vi "NI GetWaveform.vi"(0 "Acq ID In":refnum<k15>, 1 "Num Samps":i32=1000, 2 "Rcv Ring":i32, 3 "Reverse?":bool, 4 "Num Segs":i32=1, 5 "Motion Settings":T1={"No Motion?"=FALSE, "Motion System"=enum."NI 735x", "Motion Bd ID"=1, "Motion Profile"="SMAC1", "# Axis"=1, "Reverse Z axis?"=TRUE, "SMAC Axis"=0, "scan pair"=enum."y-(x) scan", "RT fps"=6.0, "Steps per mm"=[1000, 1000, 1000, 1000], "Motor Parameters"={"velocity ct/s"=[10000.0, 10000.0, 10000.0, 50000.0], "accel ct/s^2"=[50000.0, 50000.0, 50000.0, 200000.0]}, "One Way Scan"=FALSE, "Reverse One Way Scan"=FALSE, "Global Position (mm)"=[], "Plane"=0, "Distance between\nscan lines (um)"=0.0, "Distance between\nscan planes (um)"=0.0, "number of scan planes"=1, "Total steps in line"=0, "Xtra plane\ndistance  (um)"=100, "Xtra planes "=1, "Add Axis"=FALSE, "overshoot cts"=200, "BKPT Shift"=0, "Scan Start Time (ms)"=0, "ESP VISA"="GPIB::1::INSTR", "3rd Axis"=1, "GL Ref Out"=refnum, "Galil Address"=""} {"3rd Axis" items=["x", "y", "z", "w"]; "Xtra planes" min=1; "Xtra plane\ndistance  (um)" min=0; "Distance between\nscan planes (um)" format="%.2f"; "Distance between\nscan lines (um)" format="%.2f"; "SMAC Axis" items=["None"=0, "Axis 1"=1, "Axis 2"=2, "Axis 3"=3, "Axis 4"=4, "Axis 5"=5, "Axis 6"=6, "Axis 7"=7, "Axis 8"=8, "Vector Space 1"=17, "Vector Space 2"=18, "Vector Space 3"=19, "Vector Space 4"=20]; "Motion Bd ID" min=1 max=32 step=1}, 6 "Read Method":u16(ring) items=["Not used", "RT Read", "RT Save", "Scaled Voltage"], 7 "Channel":i32, 9 "error in":errorcluster, 10 "timeout":dbl=1.0, 11 "File Array":string[](array[string])=["blank"], 12 "Digitizer Settings":T5={"Digitizer delay (us) "=0.0, "rf points per line"=2048, "lines per plane"=128, "Samp Rate (Hz)"=100000000.0, "Additional dig delay (us)"=0.0, "Voltage Scale"=0.4, "Pre-Looks"=0, "Offset delay (us)"=0.0, "bits A/D"=8, "Avg Num"=1, "DigTimeOut"=5.0, "Rel Dig Delay"=0.0, "Dig Ch"=0, "LeCroyCluster"={"LeCroy Channels"=[TRUE, FALSE, FALSE, FALSE], "LC read pt offset"=0.0, "Sweep Avg"=FALSE}, "Main Digitizer"=enum."NI Digitizer", "Dig Config"=enum."Single channel", "Digitizer ID Cluster"={"Acqiris/Alazar/SP ID"=[], "NI Instr Handles"=[], "LeCroy VISA"="", "GaGe Handle"={"Handle"=0, "Sample size"=0, "Resolution"=0, "Offset"=0, "Channels"=0, "Boards"=0}, "ATS Ref"="ATS9350", "Acqiris Address"=["PCI::INSTR0"], "ADQRef"=refnum, "adq_cu_ptr"=refnum}, "Trigger Settings"={"Trig Source"=1, "Trig Coupling"=0, "Trig Slope"=0, "Level (mV)"=1500.0}, "Bulk Acq"=FALSE, "Bulk Start Indexes"=[], "Data Ref RF"=refnum, "NI ID/Channel"=[], "Total Dig CH"=1, "Xtra Ann Trig delay (us)"=10.0, "Fix Z Delay?"=FALSE, "One Way Transmission?"=FALSE, "Data Ref Log"=refnum} {"Trigger Settings"."Trig Slope" items=["Positive", "Negative"]; "Trigger Settings"."Level (mV)" format="%.2f"; "Trigger Settings"."Trig Coupling" items=["DC 1 MOhm", "AC 1 MOhm", "DC 50 Ohm", "AC 50 Ohm"]; "Trigger Settings"."Trig Source" items=["Chan 1", "External"]; "Rel Dig Delay" format="%.2f"; "DigTimeOut" format="%.2f"; "Avg Num" min=1; "Offset delay (us)" format="%.2f"; "Additional dig delay (us)" format="%.2f"; "Digitizer delay (us)" format="%.2f"}, 13 "Start Record":i32) -> (14 "Acq ID Out":refnum<k15>, 15 "Gain Array":T9(array[cluster]), 17 "Acquired Waveform16 bit":i8[][](array[numeric]), 18 "Acquired Waveform16 bit 2":i8[][](array[numeric]), 19 "error out":errorcluster)   [LabVIEW 2022 SP3]
uses:
  -DigitizerRoutines/DigitizerSettings.ctl
  -DigitizerRoutines/Digitizer.ctl
  -DigitizerRoutines/DigConfig.ctl
  -DigitizerRoutines/DigitizerID.ctl
  C:/Windows/System32/ADQAPI_dotNet_helper.dll
  Motion Controllers/NI_controller/-NI_MotionRoutines/MotionParameters.ctl
  Motion Controllers/NI_controller/-NI_MotionRoutines/MotionSys.ctl
  Motion Controllers/-MotionRoutines/ScanAxis.ctl
  Motion Controllers/-MotionRoutines/3rdAxis.ctl
  <instrlib>/niScope/Acquire/Fetch/niScope Multi Fetch Binary 8.vi
  -ScanSystem/DataHandling/ReverseDataI8.vi
  Motion Controllers/-MotionRoutines/MotionGlobals.vi
panel:
  # "Mujst convert data at output for Integers"
  # "1-D and 2-D B scan settings"
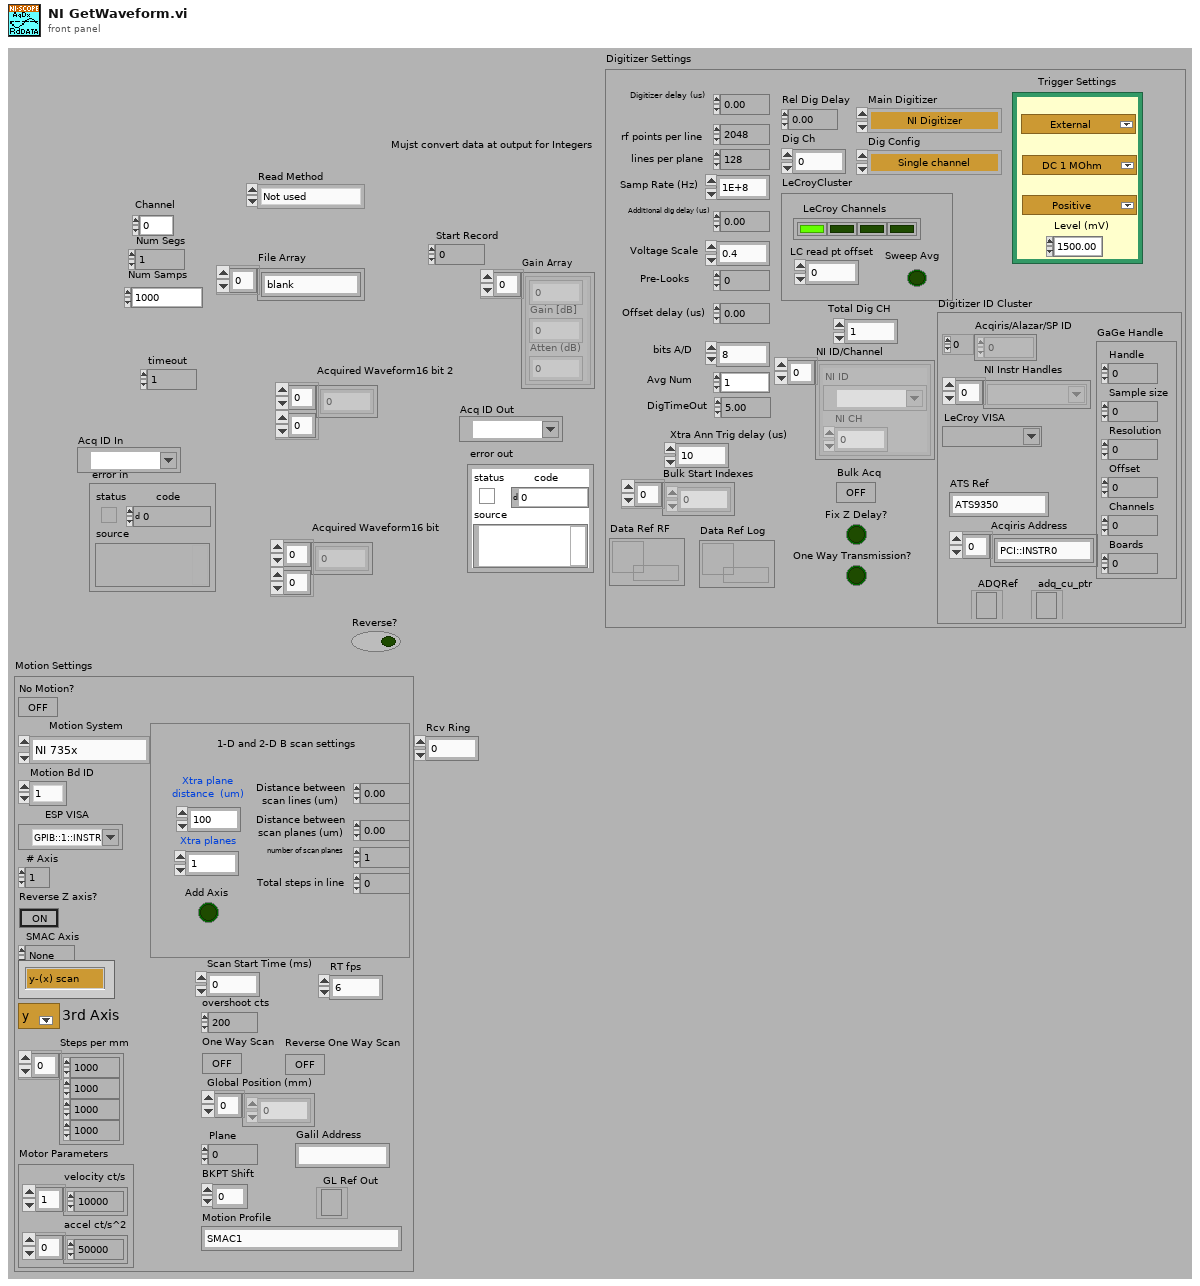
[diagram p1: front panel]
types:
  T1 = typedef "MotionParameters.ctl" = cluster{"No Motion?":bool, "Motion System":T2, "Motion Bd ID":u8, "Motion Profile":string, "# Axis":i8, "Reverse Z axis?":bool, "SMAC Axis":u16, "scan pair":T3, "RT fps":sgl, "Steps per mm":i32[], "Motor Parameters":cluster{"velocity ct/s":dbl[], "accel ct/s^2":dbl[]}, "One Way Scan":bool, "Reverse One Way Scan":bool, "Global Position (mm)":dbl[], "Plane":i32, "Distance between\nscan lines (um)":sgl, "Distance between\nscan planes (um)":sgl, "number of scan planes":i32, "Total steps in line":i32, "Xtra plane\ndistance  (um)":i32, "Xtra planes ":i32, "Add Axis":bool, "overshoot cts":i32, "BKPT Shift":i32, "Scan Start Time (ms)":u32, "ESP VISA":refnum<visa-resource-name>, "3rd Axis":T4, "GL Ref Out":refnum<k7>, "Galil Address":string}
  T2 = typedef "MotionSys.ctl" = enum16{"MM3000", "NI 735x", "Newport ESP", "No Motion Card", "Galil"}
  T3 = typedef "ScanAxis.ctl" = enum16{"y-(x) scan", "x-(y) scan", "z-(x) scan", "z-(y) scan", "y-(z) scan", "x-(z) scan", "w-(x) scan", "w-(y) scan", "w-(z) scan", "x-(w) scan", "y-(w) scan", "z-(w) scan"}
  T4 = typedef "3rdAxis.ctl" = u16
  T5 = typedef "DigitizerSettings.ctl" = cluster{"Digitizer delay (us) ":dbl, "rf points per line":i32, "lines per plane":i32, "Samp Rate (Hz)":dbl, "Additional dig delay (us)":dbl, "Voltage Scale":dbl, "Pre-Looks":i32, "Offset delay (us)":dbl, "bits A/D":i8, "Avg Num":i32, "DigTimeOut":sgl, "Rel Dig Delay":sgl, "Dig Ch":i32, "LeCroyCluster":cluster{"LeCroy Channels":bool[], "LC read pt offset":dbl, "Sweep Avg":bool}, "Main Digitizer":T6, "Dig Config":T7, "Digitizer ID Cluster":T8, "Trigger Settings":cluster{"Trig Source":u16, "Trig Coupling":u16, "Trig Slope":u16, "Level (mV)":dbl}, "Bulk Acq":bool, "Bulk Start Indexes":i32[], "Data Ref RF":refnum<data-value>, "NI ID/Channel":cluster{"NI ID":refnum<k15>, "NI CH":i32}[], "Total Dig CH":i32, "Xtra Ann Trig delay (us)":dbl, "Fix Z Delay?":bool, "One Way Transmission?":bool, "Data Ref Log":refnum<data-value>}
  T6 = typedef "Digitizer.ctl" = enum16{"Acqiris Digitizer", "NI Digitizer", "LeCroy", "GaGe", "AlazarTech", "No Digitizer", "Teledyne"}
  T7 = typedef "DigConfig.ctl" = enum16{"Single channel", "2 Chans w/ 2 Acqiris", "2 Chans w/ 1 Acqiris", "5-CH Pulser New", "5-CH pulser w/ ann array", "5-pass style ann array", "Empty"}
  T8 = typedef "DigitizerID.ctl" = cluster{"Acqiris/Alazar/SP ID":u32[], "NI Instr Handles":refnum<k15>[], "LeCroy VISA":refnum<visa-resource-name>, "GaGe Handle":cluster{"Handle":u32, "Sample size":u32, "Resolution":i32, "Offset":i32, "Channels":u32, "Boards":u32}, "ATS Ref":string, "Acqiris Address":string[], "ADQRef":refnum<k24>, "adq_cu_ptr":refnum<k24>}
  T9 = cluster{sgl, "Gain [dB]  ":sgl, "Atten (dB)":sgl}[]
  T10 = cluster{"actualSamples":i32, "absoluteInitialX":dbl, "relativeInitialX":dbl, "xIncrement":dbl, "offset":dbl, "gain":dbl, "reserved1":dbl, "reserved2":dbl}[]
  T11 = cluster{"actualSamples":i32, "absoluteInitialX":dbl, "relativeInitialX":dbl, "xIncrement":dbl, "offset":dbl, "gain":dbl, "reserved1":dbl, "reserved2":dbl}
  T12 = cluster{sgl, "Gain [dB]  ":sgl, "Atten (dB)":sgl}
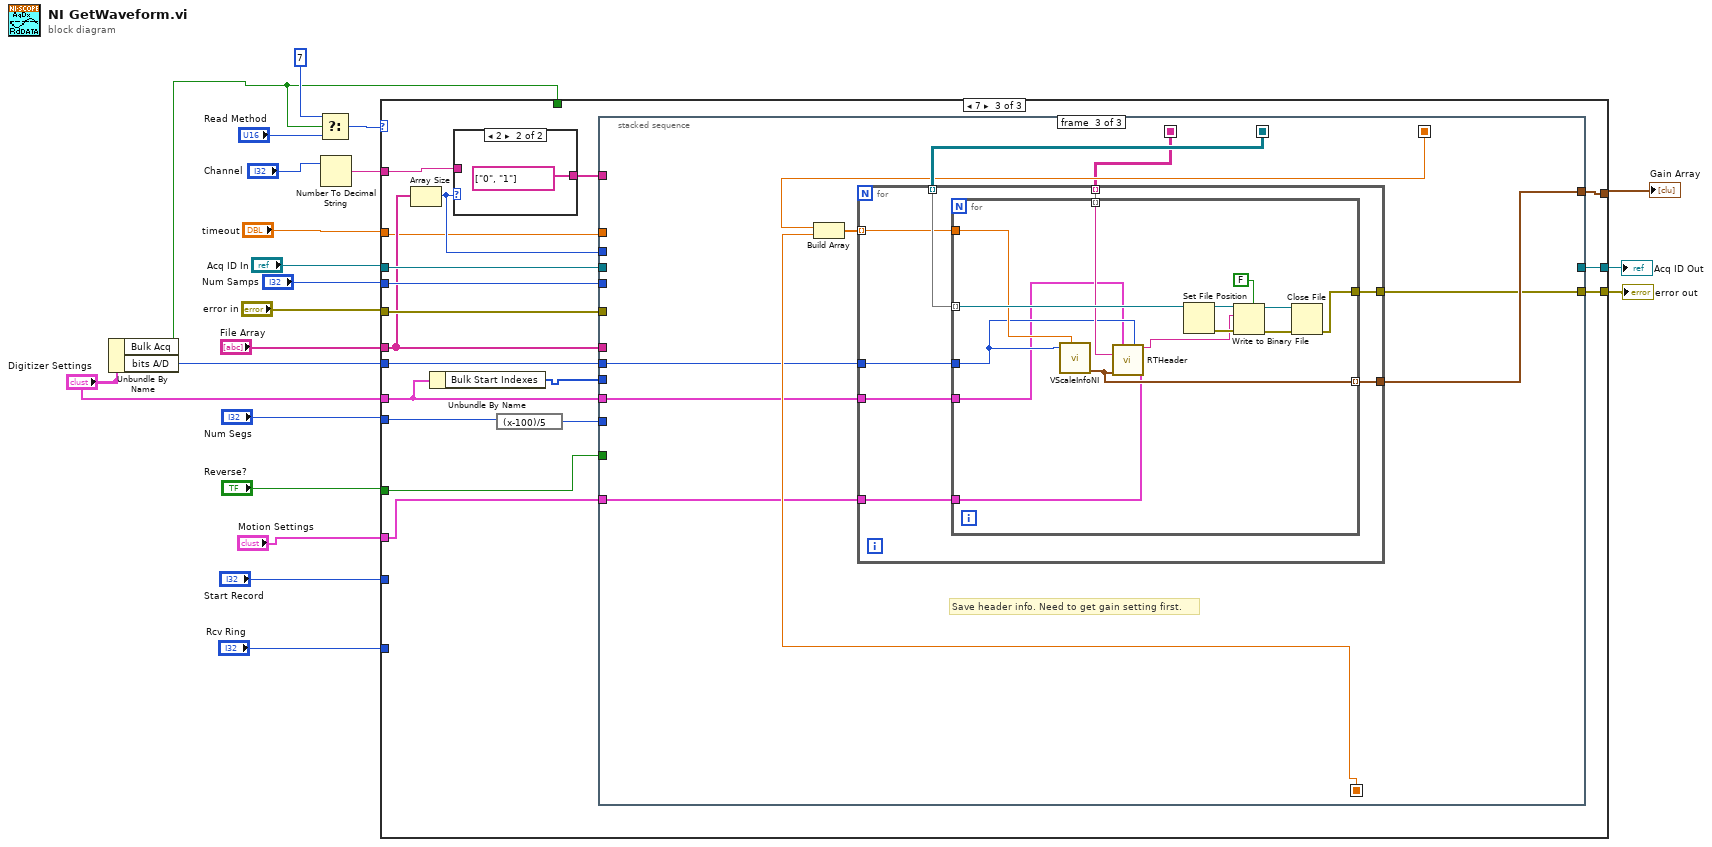
[diagram p0: block diagram]
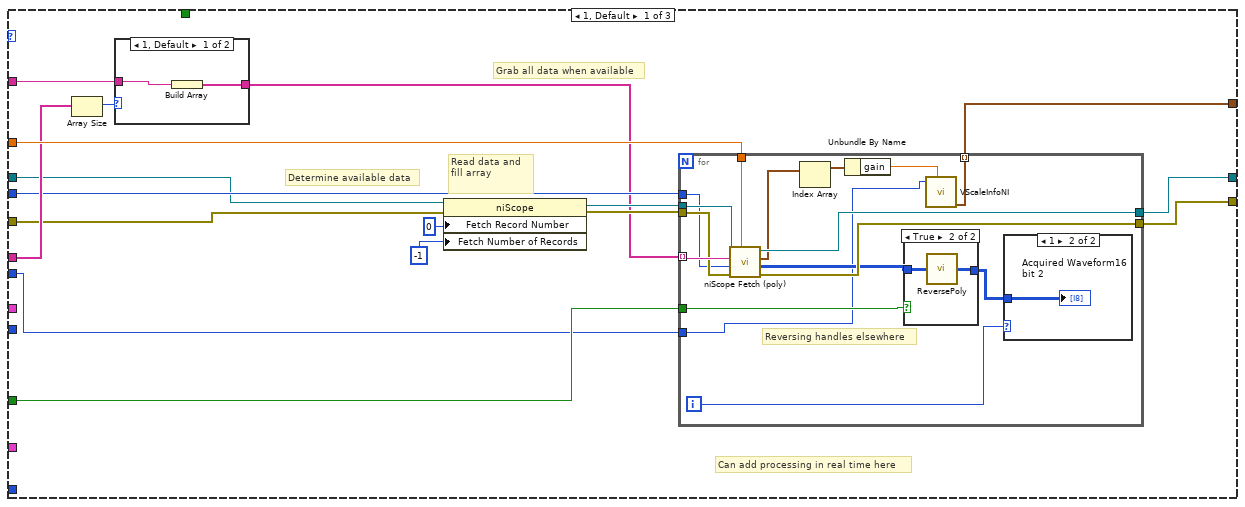
[diagram p2: hidden frame]
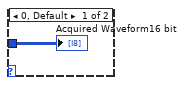
[diagram p3: hidden frame]
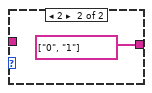
[diagram p5: hidden frame]
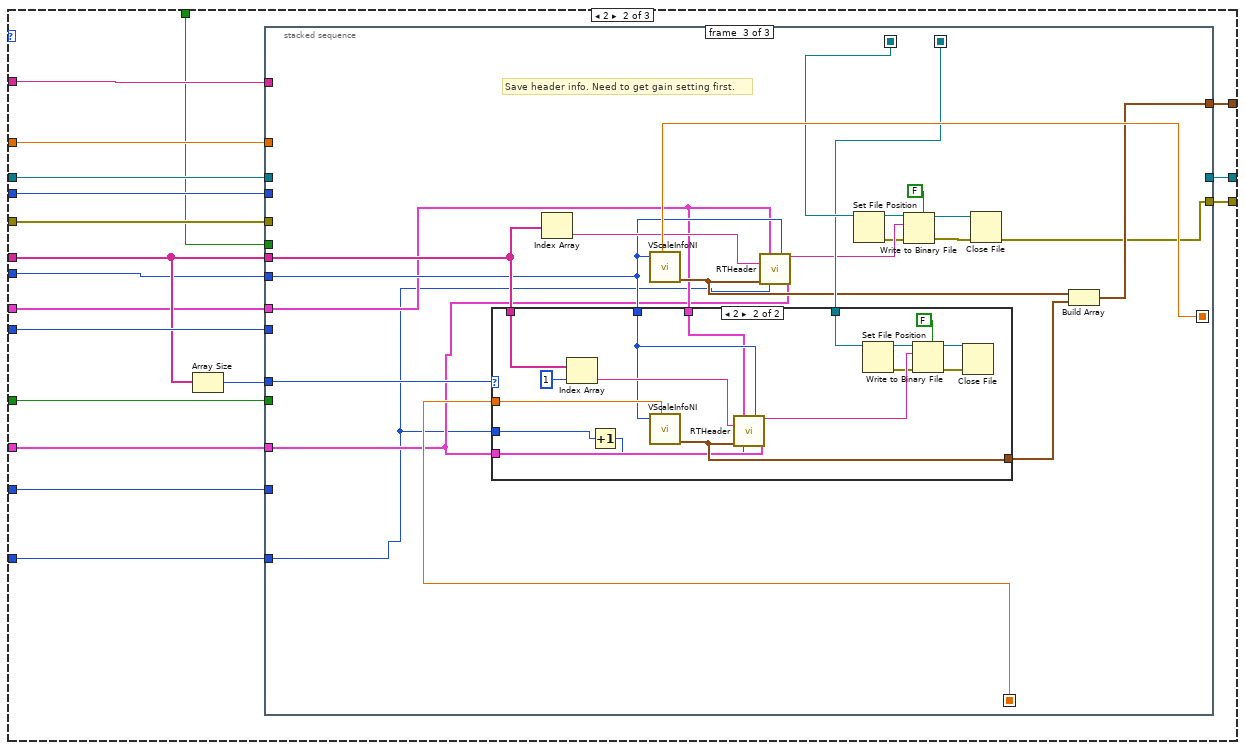
[diagram p6: hidden frame]
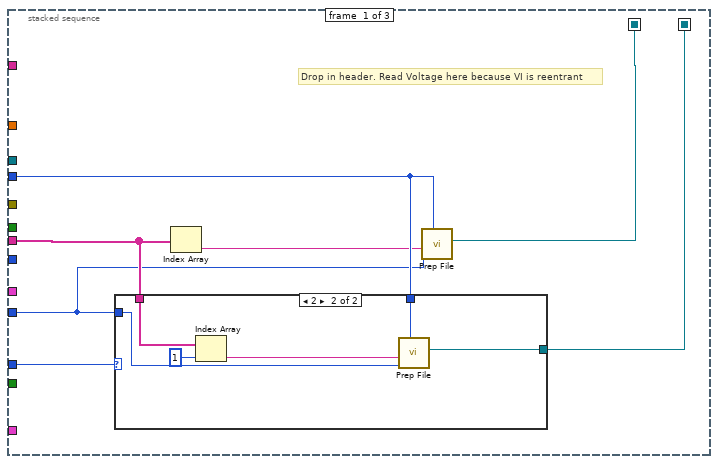
[diagram p7: hidden frame]
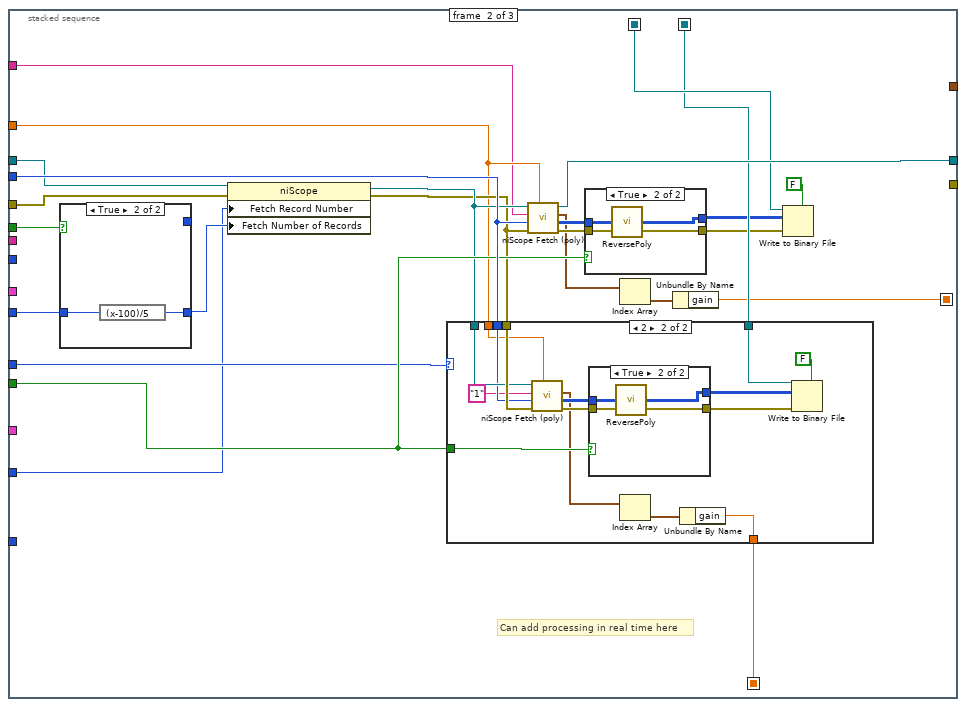
[diagram p9: hidden frame]
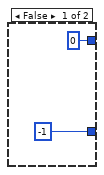
[diagram p13: hidden frame]
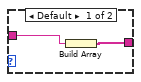
[diagram p15: hidden frame]
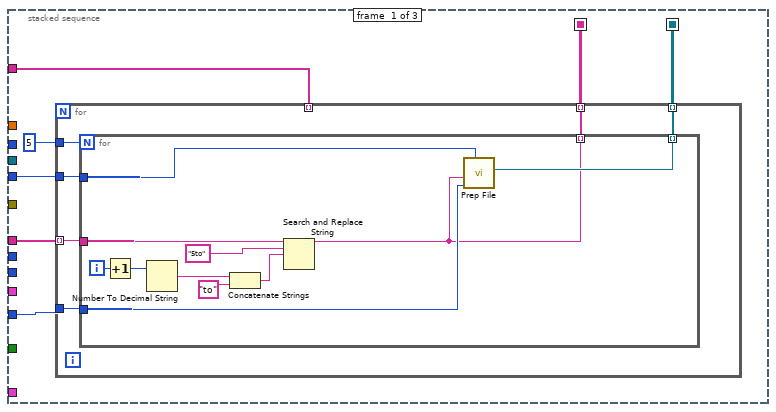
[diagram p16: hidden frame]
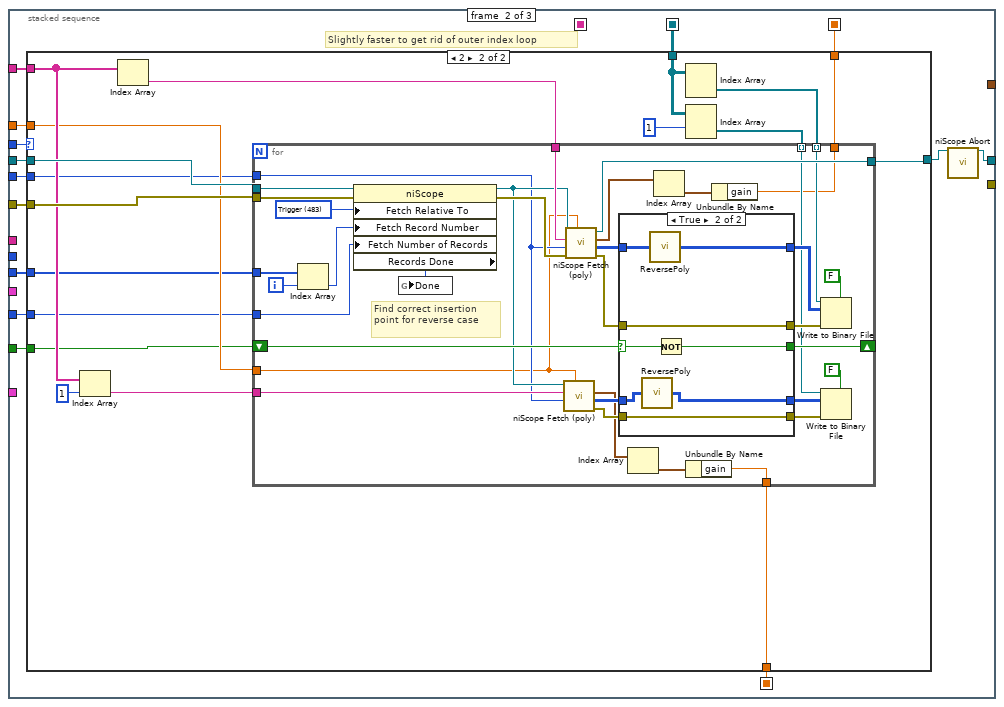
[diagram p17: hidden frame]
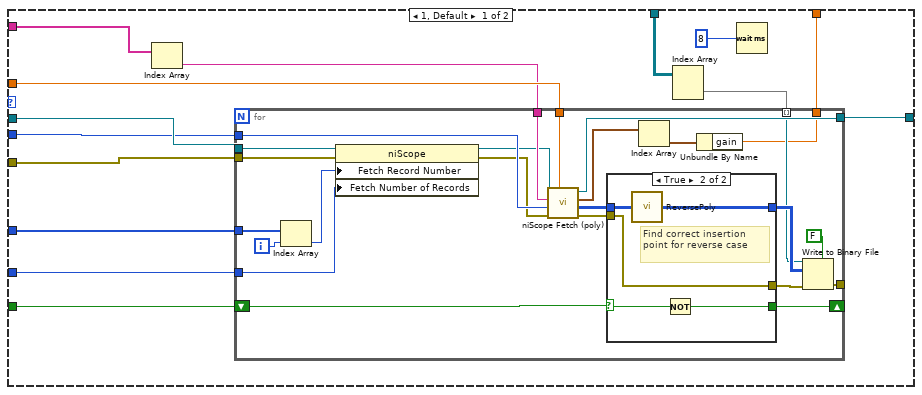
[diagram p18: hidden frame]
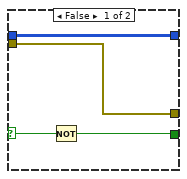
[diagram p19: hidden frame]
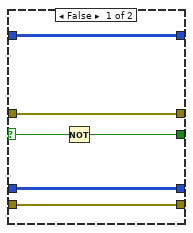
[diagram p20: hidden frame]
diagram:
  n1 = Unbundle By Name("Digitizer Settings") -> ("Bulk Acq"=w2:bool, "bits A/D"=w5:i8)
  n2 = Select(t=7, s=w2, f="Read Method") -> (s? t:f=w10:i32)
  n3 = Number To Decimal String(number="Channel") -> (decimal integer string=w12:string)  [unwired: 1 out]
  n4 = case shown="7" w10 {
    tunnel: [w26 w70 w203] -> w7
    tunnel: [w38 w80 w202] -> w15
    tunnel: "error in" -> [w29 w75 w199]
    tunnel: "Acq ID In" -> [w30 w79 w201]
    tunnel: "timeout" -> [w37 w78 w189]
    tunnel: "Num Samps" -> [w34 w77 w200]
    tunnel: "Num Segs" -> [_ w74 w194]
    tunnel: "Reverse?" -> [w23 w76 w192]
    tunnel: "File Array" -> [w36 w72 w197]
    tunnel: w12 -> [w35 w71 w196]
    tunnel: w2 -> [_ w69 _]
    tunnel: "Start Record" -> [_ w68 _]
    tunnel: [w24 w67 w191] -> w6
    tunnel: w5 -> [w22 w66 w190]
    tunnel: "Digitizer Settings" -> [_ w65 w187]
    tunnel: "Motion Settings" -> [_ w64 w188]
    tunnel: "Rcv Ring" -> [_ w63 _]
    frame 1, Default {
      # "Can add processing in real time here"
      # "Read data and fill array"
      # "Grab all data when available"
      # "Determine available data"
      n5 = Array Size(array=w36) -> (size(s)=w33:i32)
      n6 = case shown="1, Default" w33 {
        tunnel: [w61 string[] ["0", "1"] ("File Array")] -> w25
        tunnel: w35 -> [w60 _]
        frame 1, Default {
          n7 = Build Array(w60) -> (w61:string[])
        }
        frame 2 {
        }
      }
      n8 = property class="niScope"(reference=w30, error in=w29, "Fetch Record Number"=0 ("Fetch:Fetch Record Number"), "Fetch Number of Records"=-1 ("Fetch:Fetch Number of Records")) -> (reference out=w32:refnum<k15>, error out=w31:errorcluster)
      n9 = for {
        tunnel: [w49] -> w26
        tunnel: w25 -> [w54] mode=indexing
        tunnel: w37 -> [w47]
        tunnel: w32 -> [w53]
        tunnel: w31 -> [w52]
        tunnel: w34 -> [w51]
        tunnel: [w50] -> w38
        tunnel: [w48] -> w24 mode=indexing
        tunnel: w23 -> [w42]
        tunnel: w22 -> [w39]
        i -> [w40]
        # "Reversing handles elsewhere"
        n10 = call-poly <instrlib>:"niScope Fetch (poly).vi"("timeout"=w47, "error in"=w52, "numSamples"=w51, "channels"=w54, "instrument handle"=w53) -> ("error out"=w50:errorcluster, "wfm"=w43:i8[][], "wfm info"=w46:T10, "instrument handle out"=w49:refnum<k15>)  [unwired: 3 out]
        n11 = Index Array(array=w46) -> (element=w45:T11)  [unwired: 1 in]
        n12 = Unbundle By Name(w45) -> ("gain"=w44:dbl)
        n13 = case shown="True" w42 {
          tunnel: w43 -> [w57 w59]
          tunnel: [w57 w58] -> w41
          frame False {
          }
          frame True {
            n14 = call-poly "ReversePoly.vi"("Array in"=w59) -> ("Array out"=w58:i8[][])
          }
        }
        n15 = call "VScaleInfoNI.vi"("A/D bits"=w39, "gain"=w44) -> ("Voltage Scale"=w48:T12)  [unwired: 5 in, 3 out]
        n16 = case shown="1" w40 {
          tunnel: w41 -> [w55 w56]
          frame 0, Default {
            "Acquired Waveform16 bit" <- w55
          }
          frame 1 {
            "Acquired Waveform16 bit 2" <- w56
          }
        }
      }
    }
    frame 2 {
      n17 = Array Size(array=w72) -> (size(s)=w73:i32)
      n18 = stacked-sequence {
        seq-local: [w87 _ _] -> [_ w115 w166]
        seq-local: [w82 _ _] -> [_ w108 w165]
        seq-local: [_ w102 _] -> [_ _ w167]
        seq-local: [_ w101 _] -> [_ _ w168]
        tunnel: [_ w118 _] -> w70
        tunnel: [_ _ w160] -> w80
        tunnel: w79 -> [_ w112 _]
        tunnel: w78 -> [_ w107 _]
        tunnel: w74 -> [w84 w103 _]
        tunnel: w77 -> [w85 w117 _]
        tunnel: w72 -> [w86 _ w159]
        tunnel: w76 -> [_ w116 _]
        tunnel: w75 -> [_ w111 _]
        tunnel: w73 -> [w83 w109 w164]
        tunnel: w71 -> [_ w104 _]
        tunnel: w69 -> [_ w106 _]
        tunnel: w68 -> [_ w105 _]
        tunnel: [_ _ w161] -> w67
        tunnel: w66 -> [_ _ w151]
        tunnel: w65 -> [_ _ w150]
        tunnel: w64 -> [_ _ w149]
        tunnel: w63 -> [_ _ w148]
        frame #0 {
          # "Drop in header. Read Voltage here because VI is reentrant"
          n19 = case shown="2" w83 {
            tunnel: w86 -> [_ w92]
            tunnel: [_ w91] -> w82
            tunnel: w84 -> [_ w89]
            tunnel: w85 -> [_ w88]
            frame 0, Default {
            }
            frame 2 {
              n20 = Index Array(array=w92, index=1) -> (element=w90:string)
              n21 = call "Prep File.vi"("Num Samps"=w88, "Num Segs"=w89, "File Name"=w90) -> ("refnum out"=w91:refnum<file>)  [unwired: 4 in, 1 out]
            }
          }
          n22 = Index Array(array=w86) -> (element=w81:string)  [unwired: 1 in]
          n23 = call "Prep File.vi"("Num Samps"=w85, "Num Segs"=w84, "File Name"=w81) -> ("refnum out"=w87:refnum<file>)  [unwired: 4 in, 1 out]
        }
        frame #1 {
          # "Can add processing in real time here"
          n24 = case shown="True" w106 {
            tunnel: [0 ("Fetch:Fetch Record Number") _] -> _
            tunnel: [-1 ("Fetch:Fetch Number of Records") w147] -> w110
            tunnel: w103 -> [_ w146]
            frame False {
            }
            frame True {
              n25 = expression code="(x-100)/5"(w146) -> (w147:i32)
            }
          }
          n26 = property class="niScope"(reference=w112, error in=w111, "Fetch Record Number"=w105, "Fetch Number of Records"=w110) -> (reference out=w114:refnum<k15>, error out=w113:errorcluster)
          n27 = case shown="2" w109 {
            tunnel: w113 -> [_ w133]
            tunnel: w114 -> [_ w132]
            tunnel: w117 -> [_ w131]
            tunnel: w116 -> [_ w130]
            tunnel: w108 -> [_ w129]
            tunnel: w107 -> [_ w128]
            tunnel: [_ w119] -> w102
            frame 0, Default {
            }
            frame 2 {
              n28 = call-poly <instrlib>:"niScope Fetch (poly).vi"("timeout"=w128, "error in"=w133, "numSamples"=w131, "channels"="1", "instrument handle"=w132) -> ("error out"=w126:errorcluster, "wfm"=w127:i8[][], "wfm info"=w121:T10)  [unwired: 4 out]
              n29 = case shown="True" w130 {
                tunnel: [w135 w138] -> w122
                tunnel: w127 -> [w135 w137]
                tunnel: [w134 w136] -> w123
                tunnel: w126 -> [w134 w136]
                frame False {
                }
                frame True {
                  n30 = call-poly "ReversePoly.vi"("Array in"=w137) -> ("Array out"=w138:i8[][])
                }
              }
              n31 = Index Array(array=w121) -> (element=w120:T11)  [unwired: 1 in]
              n32 = Unbundle By Name(w120) -> ("gain"=w119:dbl)
              n33 = Write to Binary File(file (use dialog)=w129, data=w122, error in=w123, 5:FALSE ("prepend array or string size? (T)")) -> ()  [unwired: 2 in, 3 out]
            }
          }
          n34 = call-poly <instrlib>:"niScope Fetch (poly).vi"("timeout"=w107, "error in"=w113, "numSamples"=w117, "channels"=w104, "instrument handle"=w114) -> ("error out"=w96:errorcluster, "wfm"=w99:i8[][], "wfm info"=w95:T10, "instrument handle out"=w118:refnum<k15>)  [unwired: 3 out]
          n35 = case shown="True" w116 {
            tunnel: [w140 w143] -> w100
            tunnel: w99 -> [w140 w142]
            tunnel: [w139 w141] -> w97
            tunnel: w96 -> [w139 w141]
            frame False {
            }
            frame True {
              n36 = call-poly "ReversePoly.vi"("Array in"=w142) -> ("Array out"=w143:i8[][])
            }
          }
          n37 = Index Array(array=w95) -> (element=w94:T11)  [unwired: 1 in]
          n38 = Unbundle By Name(w94) -> ("gain"=w101:dbl)
          n39 = Write to Binary File(file (use dialog)=w115, data=w100, error in=w97, 5:FALSE ("prepend array or string size? (T)")) -> ()  [unwired: 2 in, 3 out]
        }
        frame #2 {
          # "Save header info. Need to get gain setting first."
          n40 = case shown="2" w164 {
            tunnel: w167 -> [_ w182]
            tunnel: w165 -> [_ w178]
            tunnel: [_ w177] -> w162
            tunnel: w159 -> [_ w175]
            tunnel: w151 -> [_ w173]
            tunnel: w150 -> [_ w172]
            tunnel: w149 -> [_ w171]
            tunnel: w148 -> [_ w170]
            frame 0, Default {
            }
            frame 2 {
              n41 = Index Array(array=w175, index=1) -> (element=w174:string)
              n42 = Increment(x=w170) -> (x+1=w169:i32)
              n43 = call "VScaleInfoNI.vi"("A/D bits"=w173, "gain"=w182) -> ("Voltage Scale"=w177:T12)  [unwired: 5 in, 3 out]
              n44 = call "RTHeader.vi"("Digitizer Settings"=w172, "Dig Word Size"=w173, "File Name In"=w174, "Votage scaling"=w177, "Pulser Channel"=w169, "Motion Settings"=w171) -> ("Header String Out"=w181:string)  [unwired: 8 in, 1 out]
              n45 = Set File Position(refnum=w178) -> (refnum out=w180:refnum<file>, error out=w179:errorcluster)  [unwired: 3 in]
              n46 = Write to Binary File(file (use dialog)=w180, data=w181, error in=w179, 5:FALSE ("prepend array or string size? (T)")) -> (refnum out=w183:refnum<file>, error out=w184:errorcluster)  [unwired: 2 in, 1 out]
              n47 = Close File(refnum=w183, error in=w184) -> ()  [unwired: 2 out]
            }
          }
          n48 = Index Array(array=w159) -> (element=w152:string)  [unwired: 1 in]
          n49 = call "VScaleInfoNI.vi"("A/D bits"=w151, "gain"=w168) -> ("Voltage Scale"=w163:T12)  [unwired: 5 in, 3 out]
          n50 = call "RTHeader.vi"("Digitizer Settings"=w150, "Dig Word Size"=w151, "File Name In"=w152, "Votage scaling"=w163, "Pulser Channel"=w148, "Motion Settings"=w149) -> ("Header String Out"=w155:string)  [unwired: 8 in, 1 out]
          n51 = Set File Position(refnum=w166) -> (refnum out=w154:refnum<file>, error out=w153:errorcluster)  [unwired: 3 in]
          n52 = Write to Binary File(file (use dialog)=w154, data=w155, error in=w153, 5:FALSE ("prepend array or string size? (T)")) -> (refnum out=w157:refnum<file>, error out=w156:errorcluster)  [unwired: 2 in, 1 out]
          n53 = Close File(refnum=w157, error in=w156) -> (error out=w160:errorcluster)  [unwired: 1 out]
          n54 = Build Array(w163, w162) -> (w161:T9)
        }
      }
    }
    frame 7 {
      n55 = Array Size(array=w197) -> (size(s)=w195:i32)
      n56 = Unbundle By Name(w187) -> ("Bulk Start Indexes"=w186:i32[])
      n57 = case shown="2" w195 {
        tunnel: [w205 string[] ["0", "1"] ("File Array")] -> w198
        tunnel: w196 -> [w204 _]
        frame Default {
          n58 = Build Array(w204) -> (w205:string[])
        }
        frame 2 {
        }
      }
      n59 = expression code="(x-100)/5"(w194) -> (w193:i32)
      n60 = stacked-sequence {
        seq-local: [w212 _ _] -> [_ w240 w368]
        seq-local: [_ w232 _] -> [_ _ w366]
        seq-local: [_ w231 _] -> [_ _ w365]
        seq-local: [w207 _ _] -> [_ _ w362]
        tunnel: [_ w233 _] -> w203
        tunnel: [_ _ w363] -> w202
        tunnel: w201 -> [_ w244 _]
        tunnel: w189 -> [_ w243 _]
        tunnel: w193 -> [w209 w238 _]
        tunnel: w198 -> [w213 w242 _]
        tunnel: w200 -> [w210 w241 _]
        tunnel: w197 -> [w211 _ _]
        tunnel: w199 -> [_ w239 _]
        tunnel: w195 -> [_ w237 _]
        tunnel: w186 -> [_ w236 _]
        tunnel: w192 -> [_ w235 _]
        tunnel: [_ _ w367] -> w191
        tunnel: w190 -> [_ _ w361]
        tunnel: w187 -> [_ _ w360]
        tunnel: w188 -> [_ _ w359]
        frame #0 {
          n61 = for {
            tunnel: w213 -> [_] mode=indexing
            tunnel: [w219] -> w212 mode=indexing
            tunnel: w211 -> [w218] mode=indexing
            tunnel: w210 -> [w217]
            tunnel: w209 -> [w216]
            tunnel: 5 -> [w215]
            tunnel: [w214] -> w207 mode=indexing
            n62 = for {
              N: w215 -> [_]
              tunnel: [w223] -> w219 mode=indexing
              tunnel: w218 -> [w225]
              tunnel: w217 -> [w222]
              tunnel: w216 -> [w221]
              tunnel: [w220] -> w214 mode=indexing
              i -> [w224]
              n63 = Increment(x=w224) -> (x+1=w227:i32)
              n64 = Number To Decimal String(number=w227) -> (decimal integer string=w228:string)  [unwired: 1 out]
              n65 = Concatenate Strings(w228, "to") -> (w230:string)
              n66 = Search and Replace String(input string=w225, search string="5to", replace string=w230) -> (result string=w220:string)  [unwired: 2 in, 6 out]
              n67 = call "Prep File.vi"("Num Samps"=w222, "Num Segs"=w221, "File Name"=w220) -> ("refnum out"=w223:refnum<file>)  [unwired: 4 in, 1 out]
            }
          }
        }
        frame #1 {
          # "Slightly faster to get rid of outer index loop"
          n68 = case shown="2" w237 {
            tunnel: [w250 w297] -> w234
            tunnel: w244 -> [w258 w307]
            tunnel: w243 -> [w257 w304]
            tunnel: w242 -> [w253 w306]
            tunnel: w241 -> [w256 w303]
            tunnel: w240 -> [w251 w301]
            tunnel: w239 -> [w255 w308]
            tunnel: w238 -> [w249 w299]
            tunnel: w236 -> [w248 w298]
            tunnel: w235 -> [w247 w296]
            tunnel: [w245 w293] -> w232
            tunnel: [_ w292] -> w231
            frame 1, Default {
              n69 = Index Array(array=w253) -> (element=w252:string)  [unwired: 1 in]
              n70 = Index Array(array=w251) -> (element=w246:refnum<file>[])  [unwired: 2 in]
              n71 = for {
                tunnel: [w282] -> w250
                tunnel: w252 -> [w281]
                tunnel: w257 -> [w280]
                tunnel: w255 -> [w272]
                tunnel: w256 -> [w276]
                tunnel: [w277] -> _
                tunnel: w258 -> [w274]
                tunnel: w249 -> [w271]
                shift-right: [w264] -> _
                shift-left: w247 -> [w268]
                tunnel: w248 -> [w267]
                tunnel: w246 -> [w263] mode=indexing
                tunnel: [w259] -> w245
                i -> [w266]
                n72 = Index Array(array=w267, index=w266) -> (element=w265:i32)
                n73 = property class="niScope"(reference=w274, error in=w272, "Fetch Record Number"=w265, "Fetch Number of Records"=w271) -> (reference out=w275:refnum<k15>, error out=w273:errorcluster)
                n74 = call-poly <instrlib>:"niScope Fetch (poly).vi"("timeout"=w280, "error in"=w273, "numSamples"=w276, "channels"=w281, "instrument handle"=w275) -> ("error out"=w269:errorcluster, "wfm"=w262:i8[][], "wfm info"=w261:T10, "instrument handle out"=w282:refnum<k15>)  [unwired: 3 out]
                n75 = case shown="True" w268 {
                  selector: w268 -> [w284 w288]
                  tunnel: [w286 w291] -> w279
                  tunnel: w262 -> [w286 w290]
                  tunnel: [w285 w289] -> w270
                  tunnel: w269 -> [w285 w289]
                  tunnel: [w283 w287] -> w264
                  frame False {
                    n76 = Not(x=w284) -> (.not. x?=w283:bool)
                  }
                  frame True {
                    # "Find correct insertion point for reverse case"
                    n77 = call-poly "ReversePoly.vi"("Array in"=w290) -> ("Array out"=w291:i8[][])
                    n78 = Not(x=w288) -> (.not. x?=w287:bool)
                  }
                }
                n79 = Index Array(array=w261) -> (element=w260:T11)  [unwired: 1 in]
                n80 = Unbundle By Name(w260) -> ("gain"=w259:dbl)
                n81 = Write to Binary File(file (use dialog)=w263, data=w279, error in=w270, 5:FALSE ("prepend array or string size? (T)")) -> (error out=w277:errorcluster)  [unwired: 1 in, 3 out]
              }
              n82 = Wait (ms)(milliseconds to wait=8) -> ()  [unwired: 1 out]
            }
            frame 2 {
              n83 = Index Array(array=w306, index=1) -> (element=w295:string)
              n84 = Index Array(array=w306) -> (element=w309:string)  [unwired: 1 in]
              n85 = Index Array(array=w301) -> (element=w302:refnum<file>[])  [unwired: 2 in]
              n86 = Index Array(array=w301, index (row)=1) -> (element=w294:refnum<file>[])  [unwired: 1 in]
              n87 = for {
                tunnel: [w344] -> w297
                tunnel: w309 -> [w343]
                tunnel: w304 -> [w323]
                tunnel: w308 -> [w336]
                tunnel: w303 -> [w324]
                tunnel: w302 -> [w316] mode=indexing
                tunnel: w307 -> [w338]
                tunnel: w299 -> [w335]
                shift-right: [w327] -> _
                shift-left: w296 -> [w332]
                tunnel: w298 -> [w330]
                tunnel: w295 -> [w326]
                tunnel: w294 -> [w317] mode=indexing
                tunnel: [w313] -> w293
                tunnel: [w310] -> w292
                i -> [w328]
                w339 = 483 items=["Start"=482, "Trigger"=483, "Pretrigger"=477, "Now"=481, "Read Pointer"=388] ("Fetch:Fetch Relative To")
                # "Find correct insertion point for reverse case"
                n88 = Index Array(array=w330, index=w328) -> (element=w329:i32)
                n89 = property class="niScope"(reference=w338, error in=w336, "Fetch Relative To"=w339, "Fetch Record Number"=w329, "Fetch Number of Records"=w335) -> (reference out=w325:refnum<k15>, error out=w337:errorcluster, "Records Done"=w331:i32)
                n90 = global write "MotionGlobals.vi" "Done"(w331) -> ()
                n91 = call-poly <instrlib>:"niScope Fetch (poly).vi"("timeout"=w323, "numSamples"=w324, "channels"=w326, "instrument handle"=w325) -> ("error out"=w318:errorcluster, "wfm"=w321:i8[][], "wfm info"=w311:T10)  [unwired: 1 in, 4 out]
                n92 = call-poly <instrlib>:"niScope Fetch (poly).vi"("timeout"=w323, "error in"=w337, "numSamples"=w324, "channels"=w343, "instrument handle"=w325) -> ("error out"=w333:errorcluster, "wfm"=w341:i8[][], "wfm info"=w314:T10, "instrument handle out"=w344:refnum<k15>)  [unwired: 3 out]
                n93 = case shown="True" w332 {
                  selector: w332 -> [w348 w355]
                  tunnel: [w350 w358] -> w342
                  tunnel: w341 -> [w350 w357]
                  tunnel: [w349 w356] -> w334
                  tunnel: w333 -> [w349 w356]
                  tunnel: [w347 w354] -> w327
                  tunnel: [w346 w351] -> w320
                  tunnel: w321 -> [w346 w352]
                  tunnel: [w345 w353] -> w319
                  tunnel: w318 -> [w345 w353]
                  frame False {
                    n94 = Not(x=w348) -> (.not. x?=w347:bool)
                  }
                  frame True {
                    n95 = call-poly "ReversePoly.vi"("Array in"=w352) -> ("Array out"=w351:i8[][])
                    n96 = call-poly "ReversePoly.vi"("Array in"=w357) -> ("Array out"=w358:i8[][])
                    n97 = Not(x=w355) -> (.not. x?=w354:bool)
                  }
                }
                n98 = Index Array(array=w311) -> (element=w312:T11)  [unwired: 1 in]
                n99 = Index Array(array=w314) -> (element=w315:T11)  [unwired: 1 in]
                n100 = Unbundle By Name(w312) -> ("gain"=w310:dbl)
                n101 = Unbundle By Name(w315) -> ("gain"=w313:dbl)
                n102 = Write to Binary File(file (use dialog)=w316, data=w342, error in=w334, 5:FALSE ("prepend array or string size? (T)")) -> ()  [unwired: 1 in, 4 out]
                n103 = Write to Binary File(file (use dialog)=w317, data=w320, error in=w319, 5:FALSE ("prepend array or string size? (T)")) -> ()  [unwired: 1 in, 4 out]
              }
            }
          }
          n104 = call <instrlib>:"niScope Abort.vi"("instrument handle"=w234) -> ("instrument handle out"=w233:refnum<k15>)  [unwired: 1 in, 13 out]
        }
        frame #2 {
          # "Save header info. Need to get gain setting first."
          n105 = Build Array(w366, w365) -> (w364:dbl[])
          n106 = for {
            tunnel: w368 -> [w376] mode=indexing
            tunnel: [w375] -> w367
            tunnel: w364 -> [w374] mode=indexing
            tunnel: [w373] -> w363
            tunnel: w362 -> [w372] mode=indexing
            tunnel: w361 -> [w371]
            tunnel: w360 -> [w370]
            tunnel: w359 -> [w369]
            n107 = for {
              tunnel: w376 -> [w387] mode=indexing
              tunnel: [w385] -> w375 mode=indexing
              tunnel: w374 -> [w384]
              tunnel: [w381] -> w373
              tunnel: w372 -> [w380] mode=indexing
              tunnel: w371 -> [w379]
              tunnel: w370 -> [w378]
              tunnel: w369 -> [w377]
              n108 = call "VScaleInfoNI.vi"("A/D bits"=w379, "gain"=w384) -> ("Voltage Scale"=w385:T12)  [unwired: 5 in, 3 out]
              n109 = call "RTHeader.vi"("Digitizer Settings"=w378, "Dig Word Size"=w379, "File Name In"=w380, "Votage scaling"=w385, "Motion Settings"=w377) -> ("Header String Out"=w389:string)  [unwired: 9 in, 1 out]
              n110 = Set File Position(refnum=w387) -> (refnum out=w388:refnum<file>, error out=w390:errorcluster)  [unwired: 3 in]
              n111 = Write to Binary File(file (use dialog)=w388, data=w389, error in=w390, 5:FALSE ("prepend array or string size? (T)")) -> (refnum out=w386:refnum<file>, error out=w382:errorcluster)  [unwired: 2 in, 1 out]
              n112 = Close File(refnum=w386, error in=w382) -> (error out=w381:errorcluster)  [unwired: 1 out]
            }
          }
        }
      }
    }
  }
  "error out" <- w15
  "Acq ID Out" <- w7
  "Gain Array" <- w6
